vi "Read Current Tab - Label.vi"(8 "error in":errorcluster, 11 "Front Panel Reference In":refnum<vi>) -> (0 "error out":errorcluster, 2 "Tab Label":string, 3 "Front Panel Reference Out":refnum<vi>)   [LabVIEW 2017, in "DTacq Plot Display Library.lvlib"]
uses:
  DTacq Plot Display Library.lvlib
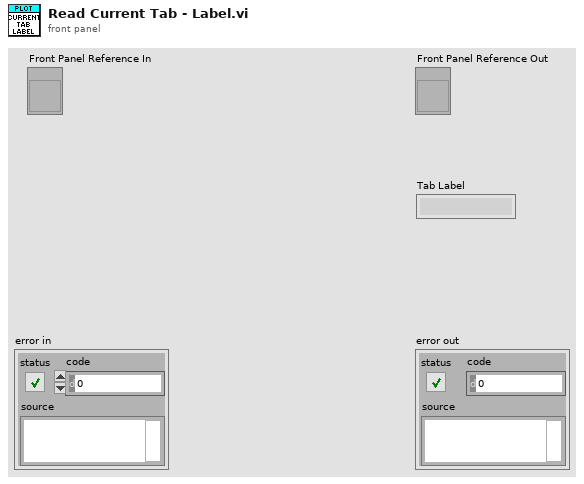
[diagram p1: front panel]
types:
  T1 = enum32{"Page 1", "Page 2", "Page 3", "Page 4", "Page 5", "Page 6"}
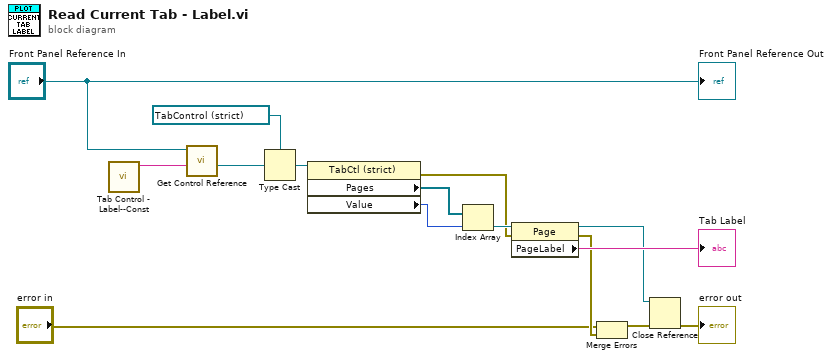
[diagram p0: block diagram]
diagram:
  n1 = call "Tab Control - Label--Const.vi"() -> ("Tab Control Label"=w13:string)  [unwired: 11 in]
  n2 = call "Get Control Reference.vi"("Control Label"=w13, "Front Panel Reference In"="Front Panel Reference In") -> ("Selected Control Reference"=w8:refnum<vi>)  [unwired: 6 in, 3 out]
  n3 = Type Cast(type=refnum<vi> refnum ("Tab Control 2"), x=w8) -> (*(type *) &x=w10:refnum<vi>)
  n4 = property class="TabCtl (strict)"(reference=w10) -> (error out=w6:errorcluster, "Pages"=w11:refnum<vi>[], "Value"=w12:T1)  [unwired: 1 in, 1 out]
  n5 = Index Array(array=w11, index=w12) -> (element=w14:refnum<vi>)
  n6 = property class="Page"(reference=w14, error in=w6) -> (reference out=w5:refnum<vi>, error out=w2:errorcluster, "PageLabel"=→"Tab Label":string)
  n7 = Merge Errors("error in", w2) -> (w3:errorcluster)
  n8 = Close Reference(reference=w5, error in (no error)=w3) -> (error out=→"error out":errorcluster)
  "Front Panel Reference Out" <- "Front Panel Reference In"
